vi "AutoMove.vi"(9 "Target Robot Angle":dbl, 10 "Distance":dbl, 11 "Movement Angle":dbl) -> (1 "Done":bool)   [LabVIEW 2017]
panel:
  in  "Turning":bool=TRUE
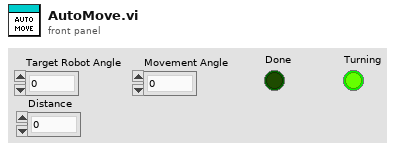
[diagram p1: front panel]
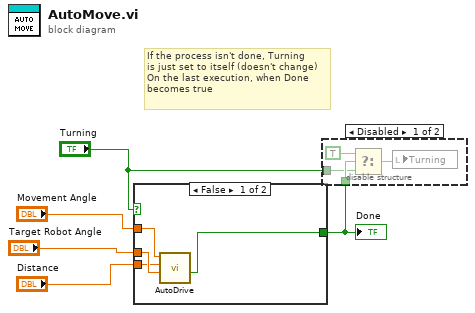
[diagram p0: block diagram]
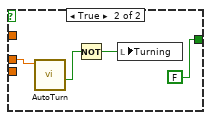
[diagram p3: hidden frame]
diagram:
  # "If the process isn't done, Turning\nis just set to itself (doesn't change)\nOn the last execution, when Done\nbecomes true"
  n1 = case shown="False" "Turning" {
    tunnel: "Target Robot Angle" -> [w9 w10]
    tunnel: "Distance" -> [w8 _]
    tunnel: "Movement Angle" -> [w7 _]
    tunnel: [w6 FALSE] -> w2
    frame False {
      n2 = call "AutoDrive.vi"("Target Robot Angle"=w9, "Distance"=w8, "Movement Angle"=w7) -> ("Done"=w6:bool)  [unwired: 8 in]
    }
    frame True {
      n3 = call "AutoTurn.vi"("Target Robot Angle"=w10) -> ("Done"=w12:bool)  [unwired: 10 in]
      n4 = Not(x=w12) -> (.not. x?=w13:bool)
      n5 = local write "Turning"(w13) -> ()
    }
  }
  "Done" <- w2
  n6 = disable-structure shown="Disabled" {
    disable-tunnel: w2 -> [w17 _]
    disable-tunnel: "Turning" -> [w15 _]
    frame Disabled {
      n7 = Select(t=TRUE, s=w17, f=w15) -> (s? t:f=w16:bool)
      n8 = local write "Turning"(w16) -> ()
    }
    frame Enabled {
    }
  }
